vi "Debug - Error Message to String.vi"(8 "error in":errorcluster) -> (0 "error out":errorcluster, 2 "Error Message":string)   [LabVIEW 2017, in "Communications Library.lvlib"]
doc: "Creates a string describing any error on the wire.\n\nReturns OK, if there is no error."
uses:
  Communications Library.lvlib
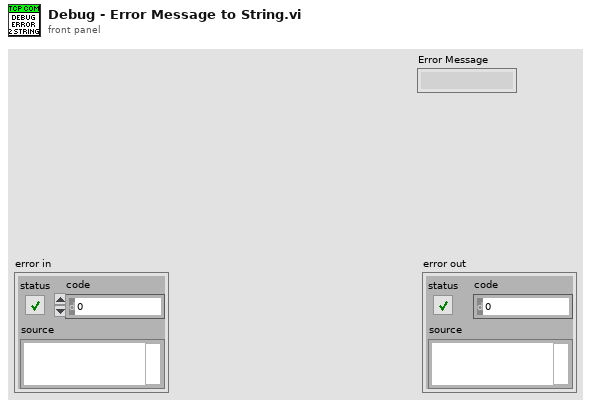
[diagram p1: front panel]
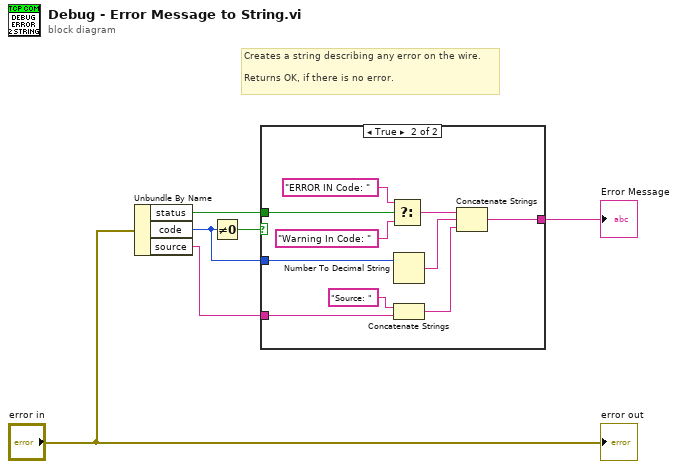
[diagram p0: block diagram]
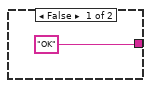
[diagram p2: hidden frame]
diagram:
  # "Creates a string describing any error on the wire.\n\nReturns OK, if there is no error."
  n1 = Unbundle By Name("error in") -> ("status"=w3:bool, "code"=w5:i32, "source"=w6:string)
  n2 = Not Equal To 0?(x=w5) -> (x != 0?=w4:bool)
  n3 = case shown="True" w4 {
    tunnel: w3 -> [_ w17]
    tunnel: w5 -> [_ w14]
    tunnel: ["OK" w8] -> w1
    tunnel: w6 -> [_ w10]
    frame False {
    }
    frame True {
      n4 = Select(t="ERROR IN Code: ", s=w17, f="Warning In Code: ") -> (s? t:f=w13:string)
      n5 = Number To Decimal String(number=w14) -> (decimal integer string=w12:string)  [unwired: 1 in]
      n6 = Concatenate Strings("Source: ", w10) -> (w9:string)
      n7 = Concatenate Strings(w13, w12, w9) -> (w8:string)
    }
  }
  "Error Message" <- w1
  "error out" <- "error in"
